vi "Read Config String.vi"(2 "key":string, 3 "section":string, 4 "Relative Path":string="..\\..\\Config files\\Default.ini") -> (0 "String":string)   [LabVIEW 2009]
uses:
  <vilib>/Utility/config.llb/Read Key (String).vi
  <vilib>/Utility/config.llb/NI_LVConfig.lvlib
panel:
  out "configuration file path":path=path "C:/Documents and Settings/Andy/Desktop/UI/Config files/Default.ini"
  out "error out":errorcluster={"status"=TRUE, "code"=7, "source"="Open Config Data.vi"}
  # "Inputs"
  # "Outputs"
  # "Locals"
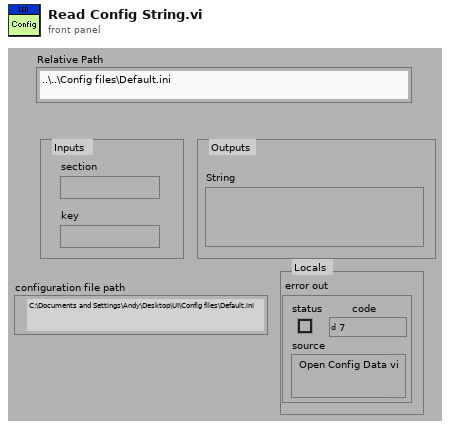
[diagram p1: front panel]
types:
  T1 = typedef "NI_LVConfig.lvlib/Config Data RefNum.ctl" = refnum<k1>
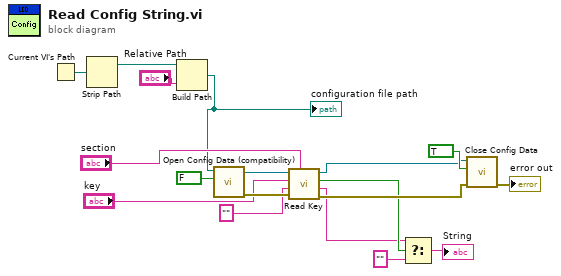
[diagram p0: block diagram]
diagram:
  n1 = Current VI's Path() -> (path=w4:path)
  n2 = Strip Path(path=w4) -> (stripped path=w2:path)  [unwired: 1 out]
  n3 = Build Path(base path=w2, name or relative path="Relative Path") -> (appended path=w1:path)
  "configuration file path" <- w1
  n4 = call <vilib>:"Open Config Data (compatibility).vi"("create file if necessary (T)"=FALSE ("create file if necessary? (T)"), "configuration file path"=w1) -> ("error out"=w14:errorcluster, "refnum"=w15:T1)  [unwired: 7 in, 1 out]
  n5 = call-poly <vilib>:"Read Key.vi"("section"="section", "error in (no error)"=w14, "default value"="" ("key 2"), "key"="key", "refnum"=w15) -> ("error out"=w12:errorcluster, "value"=w10:string, "found?"=w11:bool, "refnum out"=w5:T1)  [unwired: 1 in, 2 out]
  n6 = Select(t=w10, s=w11, f="") -> (s? t:f=→"String":string)
  n7 = call <vilib>:"Close Config Data.vi"("error in (no error)"=w12, "write file if changed (T)"=TRUE ("write configuration file? (T)"), "refnum"=w5) -> ("error out"=→"error out":errorcluster)  [unwired: 8 out]
